vi "Center text in image.vi"(6 "Text Color (red)":u32(colorbox)=16711680, 8 "error in":errorcluster, 10 "String":string, 11 "image in":T1) -> (0 "error out":errorcluster, 3 "Image Out":T1)   [LabVIEW 2013]
uses:
  <vilib>/vision/Image Controls.llb/IMAQ Image.ctl
  <resource>/objmgr/IMAQImage.rc
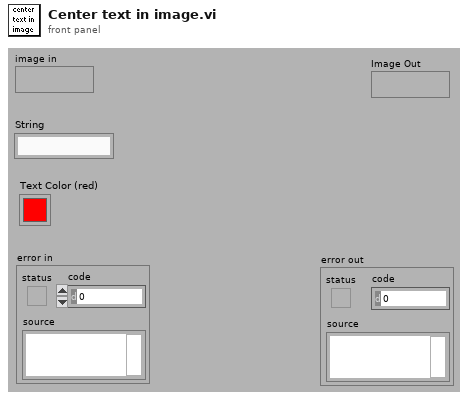
[diagram p1: front panel]
types:
  T1 = typedef "IMAQ Image.ctl" = refnum<image>
  T2 = cluster{"Desired Font (Application)":enum16{"User-specified Font", "Application Font", "System Font", "Dialog Font"}, "[User-specified Font]":cluster{"Font Name":string, "Size":i16, "Strikeout?":bool, "Italic?":bool, "Underline?":bool, "Outline?":bool, "Shadow?":bool, "Bold?":bool, "Rotation Angle":dbl}, "Horizontal Alignment":i16, "Vertical Alignment":i16}
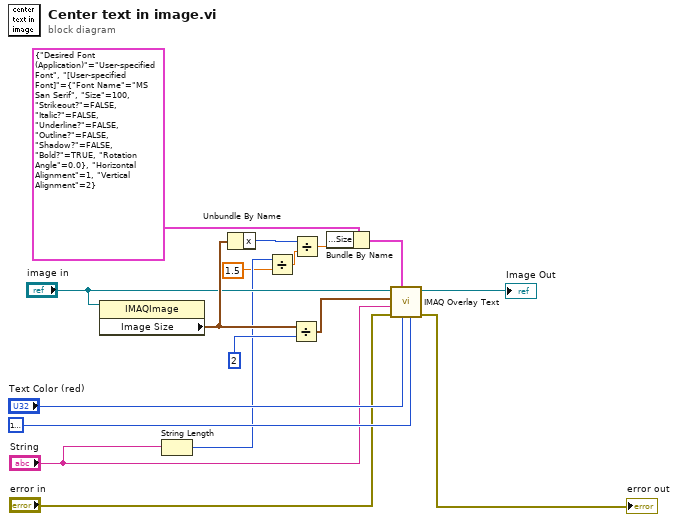
[diagram p0: block diagram]
diagram:
  n1 = property class="IMAQImage"(reference="image in") -> ("Image Size"=w13:cluster{"x":i32, "y":i32})  [unwired: 1 in, 2 out]
  n2 = String Length(string="String") -> (length=w3:i32)
  n3 = Unbundle By Name(w13) -> ("x"=w14:i32)
  n4 = Divide(x=w3, y=1.5 ("x/y")) -> (x/y=w2:dbl)
  n5 = Divide(x=w13, y=2 ("x")) -> (x/y=w11:cluster{"x":dbl, "y":dbl})
  n6 = Divide(x=w14, y=w2) -> (x/y=w15:dbl)
  n7 = Bundle By Name(cluster=T2 {"Desired Font (Application)"=enum."User-specified Font", "[User-specified Font]"={"Font Name"="MS San Serif", "Size"=100, "Strikeout?"=FALSE, "Italic?"=FALSE, "Underline?"=FALSE, "Outline?"=FALSE, "Shadow?"=FALSE, "Bold?"=TRUE, "Rotation Angle"=0.0}, "Horizontal Alignment"=1, "Vertical Alignment"=2} ("Font, Size & Style"), "[User-specified Font].Size"=w15) -> (w16:T2)
  n8 = call "IMAQ Overlay Text"("BG Color (Transparent)"=u32 16777216, "Text Color (black)"="Text Color (red)", "Font, Size & Style"=w16, "error in (no error)"="error in", "String"="String", "Origin"=w11, "Image"="image in") -> ("error out"=→"error out":errorcluster, "Image Out"=→"Image Out":T1)  [unwired: 3 in]
